vi "Fetch Measurement (Spectrum Emissions).vi"(8 "error in (no error)":errorcluster, 9 "Timeout (20000 ms)":i32=20000, 10 "Measurement Type (1)":i32=1, 11 "VISA resource name":refnum<visa-resource-name>) -> (0 "error out":errorcluster, 2 "Measured Values":dbl[](array[numeric]) format="%#.6g", 3 "VISA resource name out":refnum<visa-resource-name>)   [LabVIEW 2014, in "Agilent ESA PSA Series.lvlib"]
doc: "Returns the results of the last measurement(Spectrum Emissions) and does not initiate data acquisition."
uses:
  Agilent ESA PSA Series.lvlib
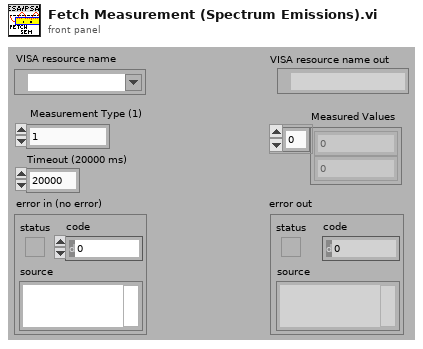
[diagram p1: front panel]
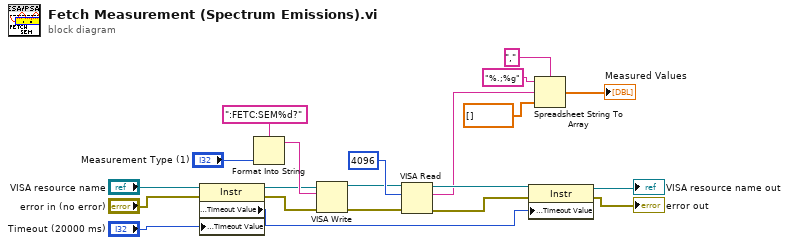
[diagram p0: block diagram]
diagram:
  n1 = property on="Property Node" class="Instr"(reference="VISA resource name", error in="error in (no error)", "General Settings:Timeout Value"="Timeout (20000 ms)") -> (reference out=w12:refnum<visa-resource-name>, error out=w13:errorcluster, "General Settings:Timeout Value"=w7:u32)
  n2 = Format Into String(format string=":FETC:SEM%d?", "Measurement Type (1)") -> (resulting string=w19:string)  [unwired: 2 in, 1 out]
  n3 = VISA Write(VISA resource name=w12, write buffer=w19, error in (no error)=w13) -> (VISA resource name out=w16:refnum<visa-resource-name>, error out=w17:errorcluster)  [unwired: 1 out]
  n4 = VISA Read(VISA resource name=w16, byte count=u32 4096, error in (no error)=w17) -> (VISA resource name out=w11:refnum<visa-resource-name>, read buffer=w2:string, error out=w8:errorcluster)  [unwired: 1 out]
  n5 = property on="Property Node" class="Instr"(reference=w11, error in=w8, "General Settings:Timeout Value"=w7) -> (reference out=→"VISA resource name out":refnum<visa-resource-name>, error out=→"error out":errorcluster)
  n6 = Spreadsheet String To Array(delimiter (Tab)=",", format string="%.;%g", spreadsheet string=w2, array type (2D Dbl)=dbl[] []) -> (array=→"Measured Values":dbl[])
